vi "Crosswalk w Button.vi"() -> ()   [LabVIEW 2023]
uses:
  7ca96a12-ef77-a741-9fb6-f6e130ed0d57.vi
  091f0f9f-ba83-5e49-bf52-7e477d967a4d.vi
  d659d5ff-7f8d-c243-b84f-b5b872c13efc.vi
  04fc8c90-0391-3c46-9268-aa9e1964be30.vi
  <extravilib>/ChannelInstances/One Element Stream-u16/Read With Abort.vi
  <extravilib>/ChannelInstances/One Element Stream-u16/Write With Abort.vi
  <extravilib>/ChannelInstances/One Element Stream-bool/Write With Abort.vi
  <extravilib>/ChannelInstances/One Element Stream-bool/Read With Abort.vi
  <extravilib>/ChannelInstances/Tag-bool/Read With Abort.vi
  <extravilib>/ChannelInstances/Tag-bool/Write With Abort.vi
  <extravilib>/ChannelInstances/Tag-bool/Instantiate.vi
  <extravilib>/ChannelInstances/Tag-bool/EndpointRead.vi
  <extravilib>/ChannelInstances/Tag-bool/Endpoint.vi
  <extravilib>/ChannelInstances/One Element Stream-bool/Instantiate.vi
  <extravilib>/ChannelInstances/One Element Stream-u16/Instantiate.vi
  <extravilib>/ChannelInstances/One Element Stream-u16/EndpointRead.vi
  <extravilib>/ChannelInstances/One Element Stream-u16/Endpoint.vi
  <extravilib>/ChannelInstances/One Element Stream-bool/Endpoint.vi
  <extravilib>/ChannelInstances/One Element Stream-bool/EndpointRead.vi
  <extravilib>/ChannelInstances/One Element Stream-bool.lvlib
  <extravilib>/ChannelInstances/One Element Stream-u16.lvlib
  <extravilib>/ChannelInstances/Tag-bool.lvlib
panel:
  out "cross pending":bool
  in  "cross":bool
  out "ped":u16(ring)
  out "light":u16(ring)
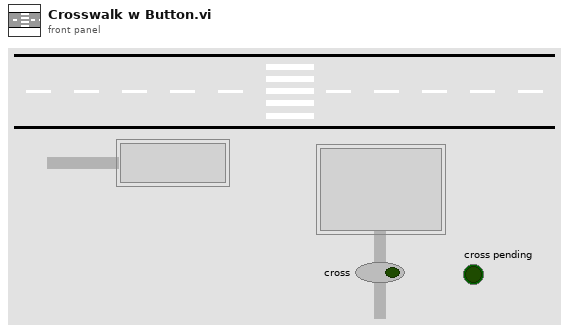
[diagram p1: front panel]
types:
  T1 = typedef "Tag-bool.lvlib/))Channel.ctl" = refnum<queue>
  T2 = typedef "One Element Stream-u16.lvlib/)Channel.ctl" = refnum<queue>
  T3 = typedef "One Element Stream-bool.lvlib/)Channel.ctl" = refnum<queue>
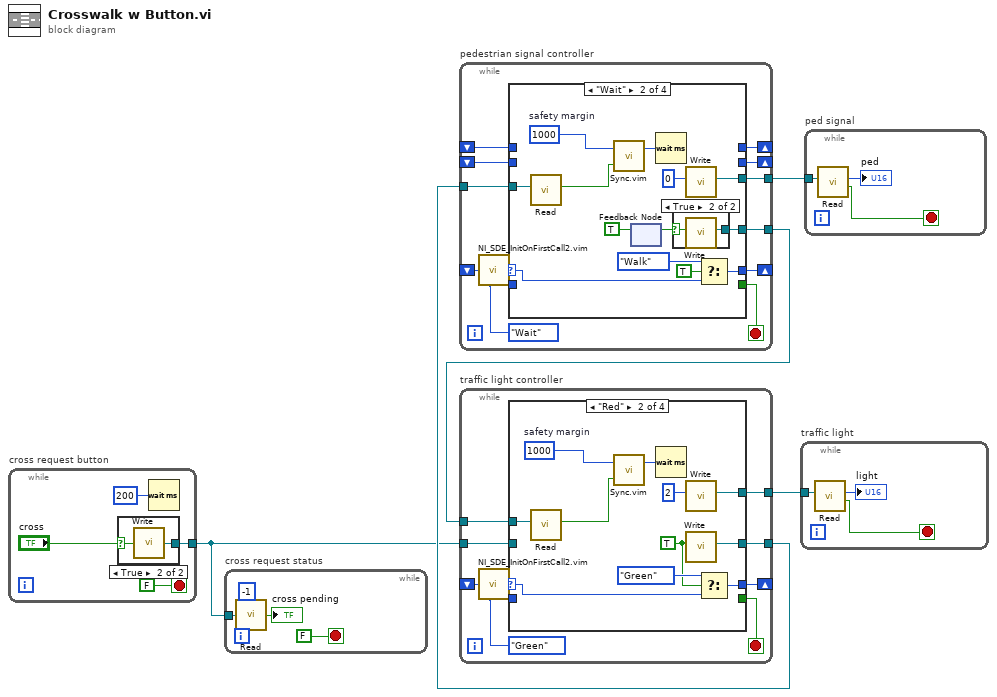
[diagram p0: block diagram]
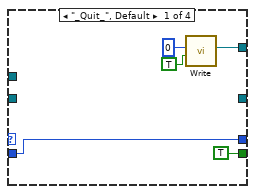
[diagram p2: hidden frame]
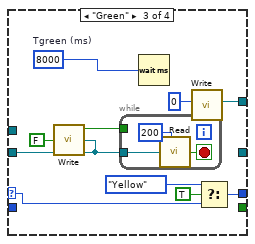
[diagram p3: hidden frame]
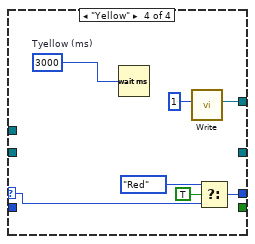
[diagram p4: hidden frame]
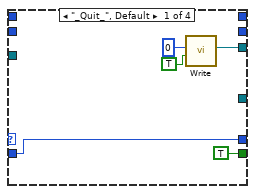
[diagram p6: hidden frame]
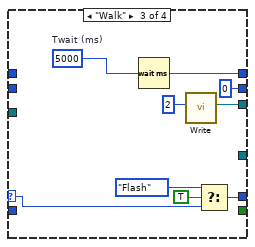
[diagram p8: hidden frame]
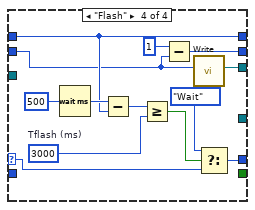
[diagram p9: hidden frame]
diagram:
  n1 = while "cross request button" {
    tunnel: [w6] -> w1
    stop <- FALSE stop-if-true
    n2 = case shown="True" "cross" {
      selector: "cross" -> [_ w11]
      tunnel: [_ w10] -> w6
      frame False {
      }
      frame True {
        n3 = call <extravilib>:"Write.vi"("element"=w11) -> ("channel"=w10:T1)  [unwired: 1 out]
      }
    }
    n4 = Wait (ms)(milliseconds to wait=u32 200) -> ()  [unwired: 1 out]
  }
  n5 = while "cross request status" {
    tunnel: w1 -> [w12]
    stop <- FALSE stop-if-true
    n6 = call <extravilib>:"Read.vi"("channel"=w12, "timeout in ms (0)"=-1) -> ("element"=→"cross pending":bool)  [unwired: 1 out]
  }
  n7 = while "pedestrian signal controller" {
    tunnel: w2 -> [w26]
    shift-right: [w25] -> _
    shift-left: _ -> [w24]
    tunnel: [w23] -> w5
    shift-right: [w22] -> _
    shift-left: _ -> [w21]
    tunnel: [w20] -> w3
    shift-right: [w17] -> _
    shift-left: _ -> [w18]
    stop <- w27 stop-if-true
    w19 = enum16{"_Quit_", "Wait", "Walk", "Flash"}."Wait"
    n8 = call "NI_SDE_InitOnFirstCall2.vim"("input"=w18, "master enum"=w19) -> ("output enum"=w16:enum16{"_Quit_", "Wait", "Walk", "Flash"})  [unwired: 1 in]
    n9 = case shown="\"Wait\"" w16 {
      selector: w16 -> [_ w45 w56 w69]
      tunnel: [TRUE _ _ _] -> w27
      tunnel: [w28 w44 w55 w68] -> w17
      tunnel: w26 -> [_ w42 _ _]
      tunnel: [_ _ w51 w62] -> w25
      tunnel: w24 -> [_ _ _ w62]
      tunnel: [w30 w40 w49 w61] -> w23
      tunnel: [_ _ u16 0 w59] -> w22
      tunnel: w21 -> [_ _ _ w58]
      tunnel: [_ w39 _ _] -> w20
      tunnel: w19 -> [w28 _ _ _]
      frame "_Quit_", Default {
        n10 = call <extravilib>:"Write.vi"("last element? (F)"=TRUE, "element"=u16 0) -> ("channel"=w30:T2)  [unwired: 8 in, 1 out]
      }
      frame "Wait" {
        w36 = u32 1000  # safety margin
        n11 = call <extravilib>:"Read.vi"("channel"=w42) -> ("element"=w37:bool)  [unwired: 7 in, 3 out]
        n12 = call "Sync.vim"("a"=w36, "b"=w37) -> ("a'"=w35:u32)  [unwired: 24 in, 1 out]
        n13 = feedback-in #1(TRUE) -> ()
        n14 = feedback #1() -> (w33:bool)  [unwired: 1 in]
        n15 = Wait (ms)(milliseconds to wait=w35) -> ()  [unwired: 1 out]
        n16 = case shown="True" w33 {
          selector: w33 -> [_ w46]
          tunnel: [_ w47] -> w39
          frame False {
          }
          frame True {
            n17 = call <extravilib>:"Write.vi"("element"=w46) -> ("channel"=w47:T3)  [unwired: 9 in, 1 out]
          }
        }
        n18 = call <extravilib>:"Write.vi"("element"=u16 0) -> ("channel"=w40:T2)  [unwired: 9 in, 1 out]
        n19 = Select(t=enum16{"_Quit_", "Wait", "Walk", "Flash"}."Walk", s=TRUE, f=w45) -> (s? t:f=w44:enum16{"_Quit_", "Wait", "Walk", "Flash"})
      }
      frame "Walk" {
        w53 = u32 5000  # Twait (ms)
        n20 = Wait (ms)(milliseconds to wait=w53) -> (millisecond timer value=w51:u32)
        n21 = call <extravilib>:"Write.vi"("element"=u16 2) -> ("channel"=w49:T2)  [unwired: 9 in, 1 out]
        n22 = Select(t=enum16{"_Quit_", "Wait", "Walk", "Flash"}."Flash", s=TRUE, f=w56) -> (s? t:f=w55:enum16{"_Quit_", "Wait", "Walk", "Flash"})
      }
      frame "Flash" {
        w63 = u32 3000  # Tflash (ms)
        n23 = Wait (ms)(milliseconds to wait=u32 500) -> (millisecond timer value=w65:u32)
        n24 = Subtract(x=w65, y=w62) -> (x-y=w64:u32)
        n25 = Greater Or Equal?(x=w64, y=w63) -> (x >= y?=w57:bool)
        n26 = Subtract(x=u16 1, y=w58) -> (x-y=w59:u16)
        n27 = call <extravilib>:"Write.vi"("element"=w58) -> ("channel"=w61:T2)  [unwired: 9 in, 1 out]
        n28 = Select(t=enum16{"_Quit_", "Wait", "Walk", "Flash"}."Wait", s=w57, f=w69) -> (s? t:f=w68:enum16{"_Quit_", "Wait", "Walk", "Flash"})
      }
    }
  }
  n29 = while "traffic light controller" {
    tunnel: w3 -> [w77]
    tunnel: [w76] -> w4
    tunnel: [w75] -> w2
    tunnel: w1 -> [w74]
    shift-right: [w72] -> _
    shift-left: _ -> [w71]
    stop <- w78 stop-if-true
    w73 = enum16{"_Quit_", "Red", "Green", "Yellow"}."Green"
    n30 = call "NI_SDE_InitOnFirstCall2.vim"("input"=w71, "master enum"=w73) -> ("output enum"=w70:enum16{"_Quit_", "Red", "Green", "Yellow"})  [unwired: 1 in]
    n31 = case shown="\"Red\"" w70 {
      selector: w70 -> [_ w94 w95 w114]
      tunnel: [TRUE _ _ _] -> w78
      tunnel: [w79 w93 w104 w113] -> w72
      tunnel: w77 -> [_ w91 _ _]
      tunnel: [w81 w89 w99 w111] -> w76
      tunnel: [_ w88 _ _] -> w75
      tunnel: [_ _ w98 _] -> w74
      tunnel: w73 -> [w79 _ _ _]
      frame "_Quit_", Default {
        n32 = call <extravilib>:"Write.vi"("last element? (F)"=TRUE, "element"=u16 0) -> ("channel"=w81:T2)  [unwired: 8 in, 1 out]
      }
      frame "Red" {
        w85 = u32 1000  # safety margin
        w87 = TRUE
        n33 = call <extravilib>:"Read.vi"("channel"=w91) -> ("element"=w86:bool)  [unwired: 7 in, 3 out]
        n34 = call "Sync.vim"("a"=w85, "b"=w86) -> ("a'"=w84:u32)  [unwired: 24 in, 1 out]
        n35 = Wait (ms)(milliseconds to wait=w84) -> ()  [unwired: 1 out]
        n36 = call <extravilib>:"Write.vi"("element"=u16 2) -> ("channel"=w89:T2)  [unwired: 9 in, 1 out]
        n37 = call <extravilib>:"Write.vi"("element"=w87) -> ("channel"=w88:T3)  [unwired: 9 in, 1 out]
        n38 = Select(t=enum16{"_Quit_", "Red", "Green", "Yellow"}."Green", s=w87, f=w94) -> (s? t:f=w93:enum16{"_Quit_", "Red", "Green", "Yellow"})
      }
      frame "Green" {
        w102 = u32 8000  # Tgreen (ms)
        n39 = call <extravilib>:"Write.vi"("element"=FALSE) -> ("previous element"=w96:bool, "channel"=w98:T1)
        n40 = while {
          tunnel: w98 -> [w107]
          tunnel: w96 -> [_]
          stop <- w106 stop-if-true
          n41 = call <extravilib>:"Read.vi"("channel"=w107, "timeout in ms (0)"=200) -> ("element"=w106:bool)  [unwired: 1 out]
        }
        n42 = Wait (ms)(milliseconds to wait=w102) -> ()  [unwired: 1 out]
        n43 = call <extravilib>:"Write.vi"("element"=u16 0) -> ("channel"=w99:T2)  [unwired: 9 in, 1 out]
        n44 = Select(t=enum16{"_Quit_", "Red", "Green", "Yellow"}."Yellow", s=TRUE, f=w95) -> (s? t:f=w104:enum16{"_Quit_", "Red", "Green", "Yellow"})
      }
      frame "Yellow" {
        w108 = u32 3000  # Tyellow (ms)
        n45 = Wait (ms)(milliseconds to wait=w108) -> ()  [unwired: 1 out]
        n46 = call <extravilib>:"Write.vi"("element"=u16 1) -> ("channel"=w111:T2)  [unwired: 9 in, 1 out]
        n47 = Select(t=enum16{"_Quit_", "Red", "Green", "Yellow"}."Red", s=TRUE, f=w114) -> (s? t:f=w113:enum16{"_Quit_", "Red", "Green", "Yellow"})
      }
    }
  }
  n48 = while "traffic light" {
    tunnel: w4 -> [w117]
    stop <- w116 stop-if-true
    n49 = call <extravilib>:"Read.vi"("channel"=w117) -> ("last element?"=w116:bool, "element"=→"light":u16)  [unwired: 7 in, 2 out]
  }
  n50 = while "ped signal" {
    tunnel: w5 -> [w120]
    stop <- w118 stop-if-true
    n51 = call <extravilib>:"Read.vi"("channel"=w120) -> ("last element?"=w118:bool, "element"=→"ped":u16)  [unwired: 7 in, 2 out]
  }
